vi "loop_with_queue.vi"() -> ()   [LabVIEW 2021]
panel:
  out "Waveform Chart":dbl(graph)
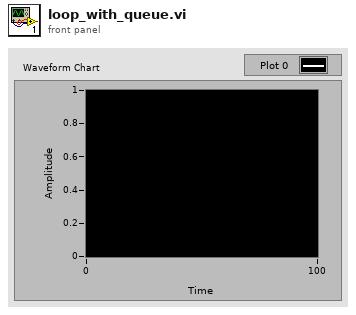
[diagram p1: front panel]
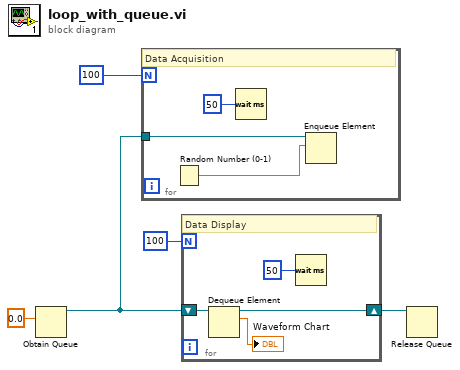
[diagram p0: block diagram]
diagram:
  n1 = Obtain Queue(element data type=0.0 ("number (0 to 1)")) -> (queue out=w2:refnum<queue>)  [unwired: 4 in, 2 out]
  n2 = for {
    N: 100 -> [_]
    tunnel: w2 -> [w7]
    # "Data Acquisition"
    n3 = Random Number (0-1)() -> (number: 0 to 1=w6:dbl)
    n4 = Wait (ms)(milliseconds to wait=u32 50) -> ()  [unwired: 1 out]
    n5 = Enqueue Element(queue=w7, element=w6) -> ()  [unwired: 2 in, 3 out]
  }
  n6 = for {
    N: 100 -> [_]
    shift-right: [w11] -> w1
    shift-left: w2 -> [w12]
    # "Data Display"
    n7 = Dequeue Element(queue=w12) -> (queue out=w11:refnum<queue>, element=→"Waveform Chart":dbl)  [unwired: 2 in, 2 out]
    n8 = Wait (ms)(milliseconds to wait=u32 50) -> ()  [unwired: 1 out]
  }
  n9 = Release Queue(queue=w1) -> ()  [unwired: 2 in, 3 out]
